vi "Top-Level.vi"() -> ()   [LabVIEW 2011]
uses:
  <vilib>/Platform/TimedLoop/XDataNode/timing_clust.ctl
  <vilib>/Platform/TimedLoop/XDataNode/nitl_modes.ctl
  <vilib>/Platform/TimedLoop/XDataNode/wakeup.ctl
  <vilib>/rvi/eio/common/nirviEmuTemplateMethod_errors.vi
  <vilib>/eio/EIONode/EIONode.xnode
  <vilib>/Platform/TimedLoop/XDataNode/XDataNode.xnode
  <vilib>/Platform/TimedLoop/XDataNode/XDNodeRunTimeDep.lvlib
panel:
  in  "manual steering":bool
  out "Velocity counts":u32
  out "Write error?":bool
  out "Read Error?":bool
  out "CS?":bool
  out "Indicator D":u32 format="%08x"
  out "Indicator C":u32 format="%08x"
  out "Indicator B":u32 format="%08x"
  out "Indicator A":u32 format="%08x"
  out "AI3":u32 format="%08x"
  out "AI2":u32 format="%08x"
  out "AI1":u32 format="%08x"
  out "AI0":u32 format="%08x"
  in  "Enable AI15":bool
  out "AI15":u16 format="%04d"
  in  "Enable AI14":bool
  out "AI14":u16 format="%04d"
  in  "Enable AI13":bool
  out "AI13":u16 format="%04d"
  in  "Enable AI12":bool
  out "AI12":u16 format="%04d"
  in  "Enable AI11":bool
  out "AI11":u16 format="%04d"
  in  "Enable AI10":bool
  out "AI10":u16 format="%04d"
  in  "Enable AI9":bool
  out "AI9":u16 format="%04d"
  in  "Enable AI8":bool
  out "AI8":u16 format="%04d"
  in  "Enable AI7":bool
  out "AI7":u16 format="%04d"
  in  "Enable AI6":bool
  out "AI6":u16 format="%04d"
  in  "Enable AI5":bool
  out "AI5":u16 format="%04d"
  in  "Enable AI4":bool
  out "AI4":u16 format="%04d"
  in  "Enable AI3":bool
  out "AI3":u16 format="%04d"
  in  "Enable AI2":bool
  out "AI2":u16 format="%04d"
  in  "Enable AI1":bool=TRUE
  out "AI1":u16 format="%04d"
  in  "Enable AI0":bool=TRUE
  out "AI0":u16 format="%04d"
  in  "ADC Run":bool=TRUE
  out "ADC Channel List":u16 format="%016b"
  in  "ADC Reset":bool
  out "Steering ON 1e-7s":u32
  out "Go Duty":u8
  out "Go Frequency":u16
  out "microblaze\\xps_gpio_0_GPIO_IO_O_pin 2":i32
  in  "manual throttle":bool
  out "Brake":bool
  out "Reverse":bool
  out "Enable":bool
  in  "uBlaze Reset":bool
  out "PWM0 period (cycles)":u32=400000
  out "PWM0 duty (cycles)":u32=80000
  in  "Clock Frequency (Hz)":u32=40000000
  out "PWM1 period(cycles)":u32=400000
  out "PWM1 duty (cycles)":u32=80000
  in  "PWM0 frequency (Hz)":u16
  in  "PWM0 duty (100*%)":u16
  in  "PWM1 frequency (Hz)":u16
  in  "PWM1 duty (100*%)":u16
  out "Steering period (cycles)":u32=400000
  out "Steering duty (cycles)":u32=80000
  out "GO period (cycles)":u32=400000
  out "GO duty (cycles)":u32=80000
  in  "Steering frequency (Hz)":u16=50
  in  "Steering ON 1e-7s":u32=8
  in  "GO frequency (Hz)":u16=1000
  in  "GO duty (100*%)":u16
  # "uBlaze Front Panel"
  # "ADC"
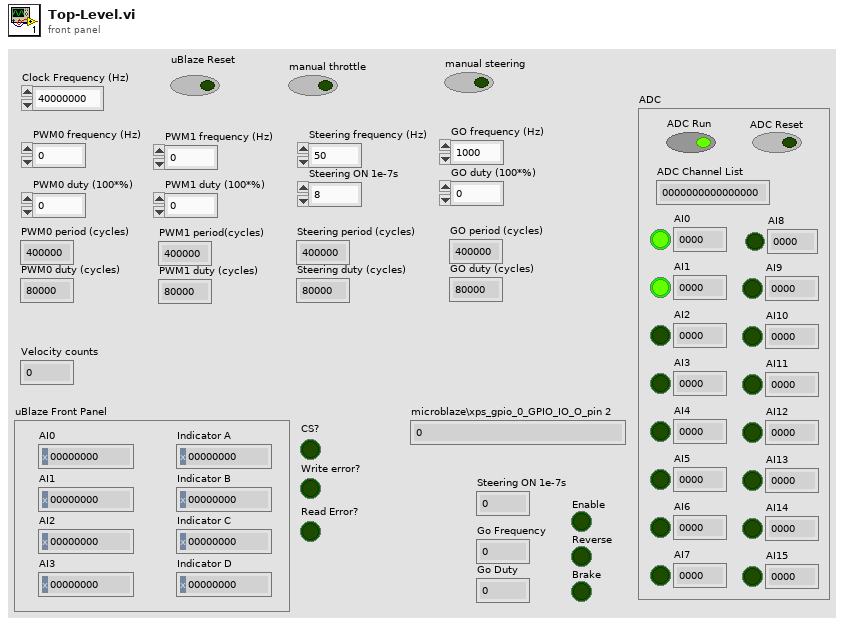
[diagram p1: front panel]
types:
  T1 = typedef "XDNodeRunTimeDep.lvlib/timing_clust.ctl" = cluster{"Expected End [f-1]":u64, "Actual End [f-1]":u64, "Finished Late? [f-1]":bool, "Expected End [i-1]":u64, "Actual End [i-1]":u64, "Finished Late? [i-1]":bool, "Expected Start [i]":u64, "Actual Start [i]":u64, "Expected Start [f]":u64, "Actual Start [f]":u64, "Source Name":string, "Structure Name":string, "Period":i64, "Deadline":i64, "Offset":i64, "Start":i64, "Priority":i32, "Timeout":i32, "Mode":T2, "Wakeup Reason":T3, "Error":errorcluster, "Source Type":string, "Secondary Source Type":string, "Global End Time":u64, "Global Start Time":u64, "Frame Duration":u64, "Iteration Duration":u64, "Assigned CPU":i32, "I/O Scan Engine Mode":u32}
  T2 = typedef "XDNodeRunTimeDep.lvlib/nitl_modes.ctl" = enum32{"No Change", "Process missed periods, maintain original phase", "Discard missed periods, maintain original phase", "Process missed periods, ignore original phase", "Discard missed periods, ignore original phase"}
  T3 = typedef "XDNodeRunTimeDep.lvlib/wakeup.ctl" = enum32{"Normal", "Aborted", "Asynchronous wakeup", "Timing source error", "Timed loop error", "Timeout"}
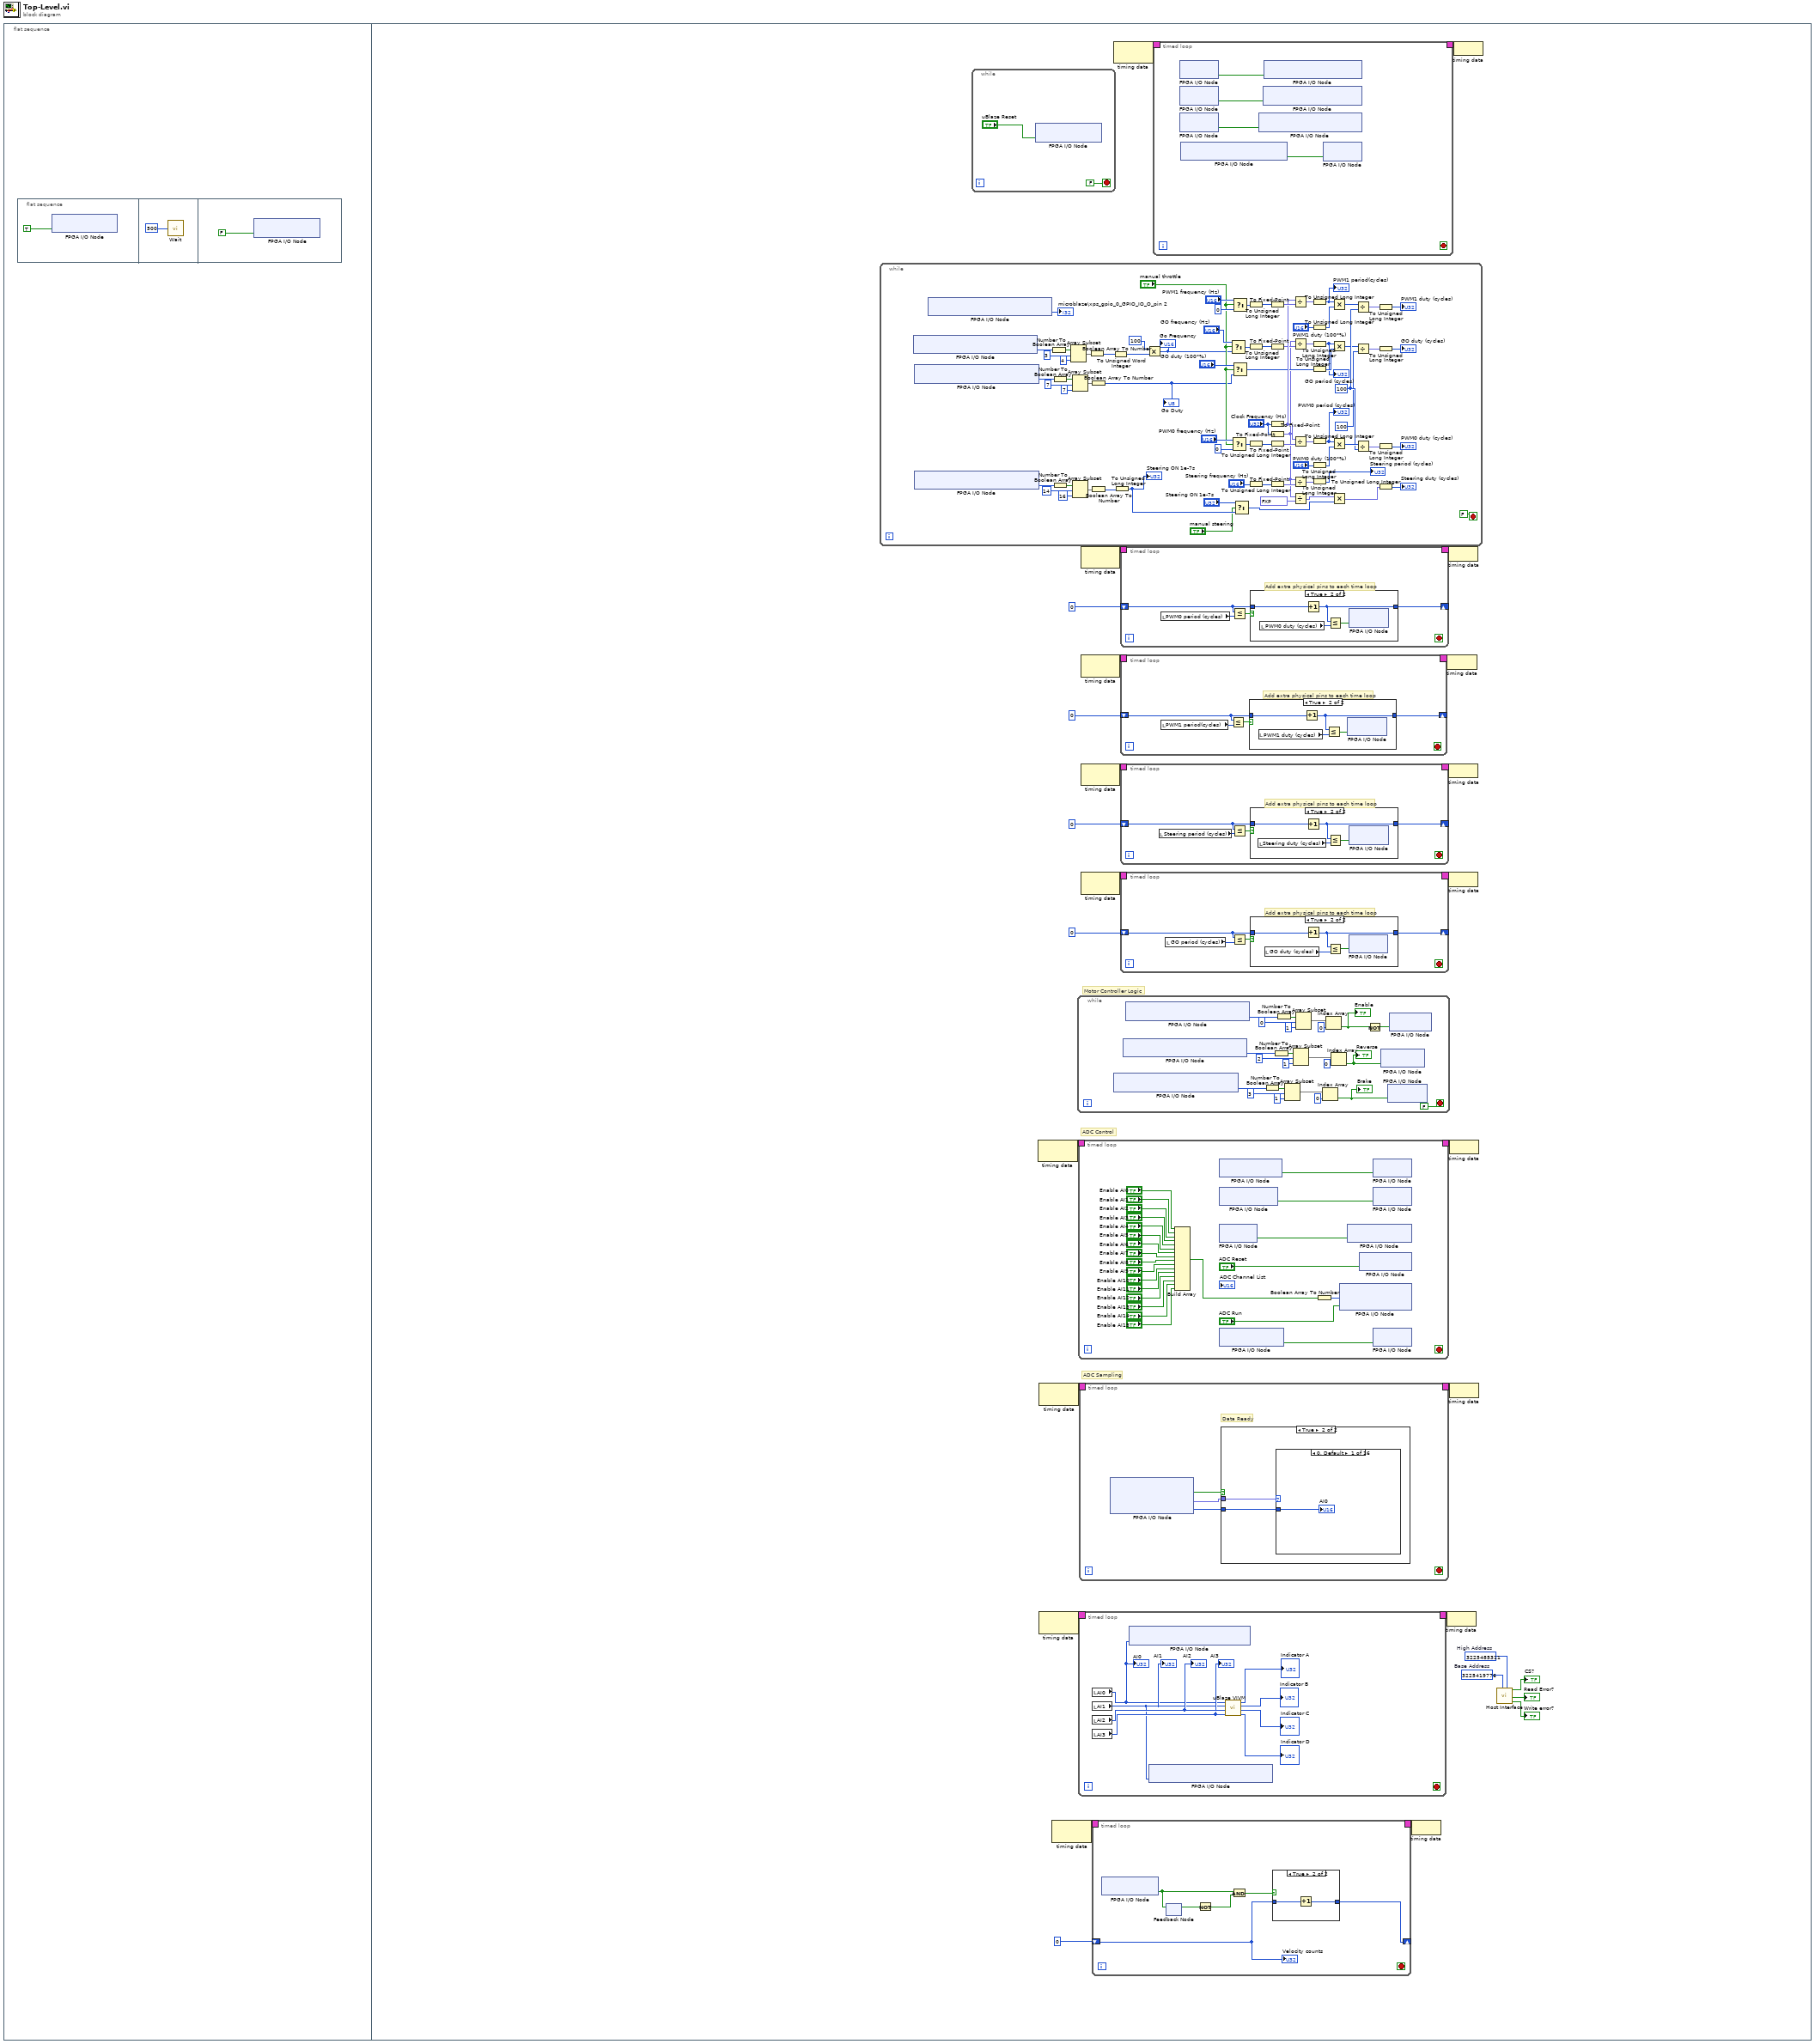
[diagram p0: block diagram]
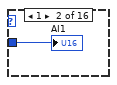
[diagram p4: hidden frame]
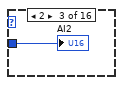
[diagram p5: hidden frame]
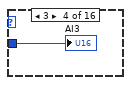
[diagram p6: hidden frame]
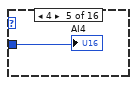
[diagram p7: hidden frame]
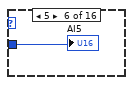
[diagram p8: hidden frame]
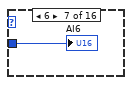
[diagram p9: hidden frame]
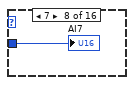
[diagram p10: hidden frame]
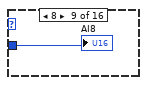
[diagram p11: hidden frame]
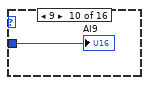
[diagram p12: hidden frame]
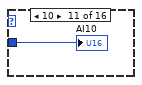
[diagram p13: hidden frame]
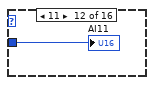
[diagram p14: hidden frame]
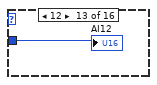
[diagram p15: hidden frame]
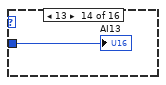
[diagram p16: hidden frame]
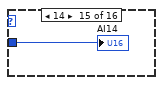
[diagram p17: hidden frame]
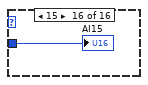
[diagram p18: hidden frame]
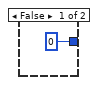
[diagram p19: hidden frame]
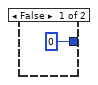
[diagram p20: hidden frame]
diagram:
  n1 = flat-sequence {
    frame #0 {
      n2 = flat-sequence {
        frame #0 {
          n3 = xnode "FPGA I/O Node"("microblaze\\reset"=TRUE ("Component-Level IP\\fpga_0_rst_1_sys_rst_pin")) -> ()  [unwired: 1 in, 1 out]
        }
        frame #1 {
          n4 = call "Wait"("Count(mSec)"=u32 500) -> ()  [unwired: 1 out]
        }
        frame #2 {
          n5 = xnode "FPGA I/O Node"("microblaze\\reset"=FALSE ("Component-Level IP\\fpga_0_rst_1_sys_rst_pin")) -> ()  [unwired: 1 in, 1 out]
        }
      }
    }
    frame #1 {
      w12 = u32 3225485311  # High Address
      w13 = u32 3225419776  # Base Address
      # "ADC Sampling"
      # "ADC Control"
      # "Motor Controller Logic"
      n6 = while {
        stop <- FALSE stop-if-true
        w191 = u32 100 ("y")
        n7 = xnode "FPGA I/O Node"() -> ("microblaze\\xps_gpio_0_GPIO_IO_O_pin"=w156:i32)  [unwired: 1 in, 1 out]
        n8 = xnode "FPGA I/O Node"() -> ("microblaze\\xps_gpio_0_GPIO_IO_O_pin"=w150:i32)  [unwired: 1 in, 1 out]
        n9 = xnode "FPGA I/O Node"() -> ("microblaze\\xps_gpio_0_GPIO_IO_O_pin"=w151:i32)  [unwired: 1 in, 1 out]
        n10 = xnode "FPGA I/O Node"() -> ("microblaze\\xps_gpio_0_GPIO_IO_O_pin"=→"microblaze\\xps_gpio_0_GPIO_IO_O_pin 2":i32)  [unwired: 1 in, 1 out]
        n11 = Number To Boolean Array(number=w156) -> (Boolean array=w160:bool[])
        n12 = Number To Boolean Array(number=w150) -> (Boolean array=w146:bool[])
        n13 = Number To Boolean Array(number=w151) -> (Boolean array=w155:bool[])
        n14 = Array Subset(array=w160, index=3, length=4) -> (w159:bool[])
        n15 = Array Subset(array=w146, index=7, length=7) -> (w147:bool[])
        n16 = Array Subset(array=w155, index=14, length=16) -> (w154:bool[])
        n17 = Boolean Array To Number(Boolean array=w159) -> (number=w143:u8)
        n18 = Boolean Array To Number(Boolean array=w147) -> (number=w145:u8)
        "Go Duty" <- w145
        n19 = Boolean Array To Number(Boolean array=w154) -> (number=w135:u16)
        n20 = To Unsigned Word Integer(number=w143) -> (unsigned 16bit integer=w142:u16)
        n21 = To Unsigned Long Integer(number=w135) -> (unsigned 32bit integer=w134:u32)
        "Steering ON 1e-7s" <- w134
        n22 = Multiply(x=u16 100, y=w142) -> (x*y=w162:u16)
        "Go Frequency" <- w162
        n23 = Select(t="GO frequency (Hz)", s="manual throttle", f=w162) -> (s? t:f=w174:u16)
        n24 = Select(t="PWM0 frequency (Hz)", s="manual throttle", f=u16 0) -> (s? t:f=w172:u16)
        n25 = Select(t="GO duty (100*%)", s="manual throttle", f=w145) -> (s? t:f=w170:u16)
        n26 = Select(t="PWM1 frequency (Hz)", s="manual throttle", f=u16 0) -> (s? t:f=w176:u16)
        n27 = Select(t="Steering ON 1e-7s", s="manual steering", f=w134) -> (s? t:f=w137:u32)
        n28 = To Unsigned Long Integer(number=w176) -> (unsigned 32bit integer=w199:u32)
        n29 = To Unsigned Long Integer(number=w174) -> (unsigned 32bit integer=w184:u32)
        n30 = To Unsigned Long Integer(number=w172) -> (unsigned 32bit integer=w203:u32)
        n31 = To Unsigned Long Integer(number="Steering frequency (Hz)") -> (unsigned 32bit integer=w186:u32)
        n32 = To Fixed-Point(number=w199) -> (fixed-point=w198:fxp<+,32,32>)  [unwired: 1 out]
        n33 = To Fixed-Point(number=w184) -> (fixed-point=w183:fxp<+,32,32>)  [unwired: 1 out]
        n34 = To Fixed-Point(number="Clock Frequency (Hz)") -> (fixed-point=w192:fxp<+,32,32>)  [unwired: 1 out]
        n35 = To Fixed-Point(number="Clock Frequency (Hz)") -> (fixed-point=w141:fxp<+,32,32>)  [unwired: 1 out]
        n36 = To Fixed-Point(number=w203) -> (fixed-point=w204:fxp<+,32,32>)  [unwired: 1 out]
        n37 = To Fixed-Point(number=w186) -> (fixed-point=w187:fxp<+,32,32>)  [unwired: 1 out]
        n38 = Divide(x=w192, y=w198) -> (x/y=w193:fxp<+,32,33>)
        n39 = Divide(x=w141, y=w183) -> (x/y=w178:fxp<+,32,33>)
        n40 = Divide(x=w192, y=w204) -> (x/y=w209:fxp<+,32,33>)
        n41 = Divide(x=w141, y=w187) -> (x/y=w189:fxp<+,32,33>)
        n42 = Divide(x=w141, y=fxp<+,32,32> 10000000.0) -> (x/y=w138:fxp<+,64,32>)
        n43 = To Unsigned Long Integer(number=w193) -> (unsigned 32bit integer=w194:u32)
        "PWM1 period(cycles)" <- w194
        n44 = To Unsigned Long Integer(number="PWM1 duty (100*%)") -> (unsigned 32bit integer=w200:u32)
        n45 = To Unsigned Long Integer(number=w178) -> (unsigned 32bit integer=w179:u32)
        "GO period (cycles)" <- w179
        n46 = To Unsigned Long Integer(number=w170) -> (unsigned 32bit integer=w185:u32)
        n47 = To Unsigned Long Integer(number=w209) -> (unsigned 32bit integer=w208:u32)
        "PWM0 period (cycles)" <- w208
        n48 = To Unsigned Long Integer(number="PWM0 duty (100*%)") -> (unsigned 32bit integer=w201:u32)
        n49 = To Unsigned Long Integer(number=w189) -> (unsigned 32bit integer=→"Steering period (cycles)":u32)
        n50 = Multiply(x=w194, y=w200) -> (x*y=w195:u32)
        n51 = Multiply(x=w179, y=w185) -> (x*y=w180:u32)
        n52 = Multiply(x=w208, y=w201) -> (x*y=w207:u32)
        n53 = Multiply(x=w138, y=w137) -> (x*y=w136:fxp<+,64,64>)
        n54 = Divide(x=w195, y=w191) -> (x/y=w196:fxp<+,32,33>)
        n55 = Divide(x=w180, y=u32 100) -> (x/y=w181:fxp<+,32,33>)
        n56 = Divide(x=w207, y=w191) -> (x/y=w206:fxp<+,32,33>)
        n57 = To Unsigned Long Integer(number=w196) -> (unsigned 32bit integer=→"PWM1 duty (cycles)":u32)
        n58 = To Unsigned Long Integer(number=w181) -> (unsigned 32bit integer=→"GO duty (cycles)":u32)
        n59 = To Unsigned Long Integer(number=w206) -> (unsigned 32bit integer=→"PWM0 duty (cycles)":u32)
        n60 = To Unsigned Long Integer(number=w136) -> (unsigned 32bit integer=→"Steering duty (cycles)":u32)
      }
      n61 = while {
        stop <- FALSE stop-if-true
        n62 = xnode "FPGA I/O Node"("microblaze\\reset"="uBlaze Reset") -> ()  [unwired: 1 in, 1 out]
      }
      n63 = node-c288() -> (w17:T1)  [unwired: 1 in]
      n64 = node-c288() -> (w8:T1)  [unwired: 1 in]
      n65 = node-c288() -> (w15:T1)  [unwired: 1 in]
      n66 = node-c288() -> (w6:T1)  [unwired: 1 in]
      n67 = while {
        stop <- FALSE stop-if-true
        n68 = xnode "FPGA I/O Node"() -> ("microblaze\\xps_gpio_0_GPIO_IO_O_pin"=w119:i32)  [unwired: 1 in, 1 out]
        n69 = xnode "FPGA I/O Node"() -> ("microblaze\\xps_gpio_0_GPIO_IO_O_pin"=w126:i32)  [unwired: 1 in, 1 out]
        n70 = xnode "FPGA I/O Node"() -> ("microblaze\\xps_gpio_0_GPIO_IO_O_pin"=w129:i32)  [unwired: 1 in, 1 out]
        n71 = Number To Boolean Array(number=w119) -> (Boolean array=w122:bool[])
        n72 = Number To Boolean Array(number=w126) -> (Boolean array=w123:bool[])
        n73 = Number To Boolean Array(number=w129) -> (Boolean array=w132:bool[])
        n74 = Array Subset(array=w122, index=3, length=1) -> (w116:bool[])
        n75 = Array Subset(array=w123, index=2, length=1) -> (w117:bool[])
        n76 = Array Subset(array=w132, index=0, length=1) -> (w113:bool[])
        n77 = Index Array(array=w116, index=0) -> (element=w114:bool)
        "Brake" <- w114
        n78 = Index Array(array=w113, index=0) -> (element=w111:bool)
        "Enable" <- w111
        n79 = Index Array(array=w117, index=0) -> (element=w115:bool)
        "Reverse" <- w115
        n80 = Not(x=w111) -> (.not. x?=w112:bool)
        n81 = xnode "FPGA I/O Node"("REVERSE"=w115) -> ()  [unwired: 1 in, 1 out]
        n82 = xnode "FPGA I/O Node"("BRAKE"=w114) -> ()  [unwired: 1 in, 1 out]
        n83 = xnode "FPGA I/O Node"("ENABLE"=w112) -> ()  [unwired: 1 in, 1 out]
      }
      n84 = timed-loop {
        timing: w17 -> [_]
        timing-out: [_] -> w16
        stop <- _ stop-if-true
        n85 = Build Array("Enable AI0", "Enable AI1", "Enable AI2", "Enable AI3", "Enable AI4", "Enable AI5", "Enable AI6", "Enable AI7", "Enable AI8", "Enable AI9", "Enable AI10", "Enable AI11", "Enable AI12", "Enable AI13", "Enable AI14", "Enable AI15") -> (w98:bool[])
        n86 = xnode "FPGA I/O Node"() -> ("ADC\\aaispics_n"=w100:bool)  [unwired: 1 in, 1 out]
        n87 = xnode "FPGA I/O Node"() -> ("ADC\\aaispiclk"=w101:bool)  [unwired: 1 in, 1 out]
        n88 = xnode "FPGA I/O Node"() -> ("SDO"=w102:bool)  [unwired: 1 in, 1 out]
        n89 = xnode "FPGA I/O Node"() -> ("ADC\\aaispimosi"=w103:bool)  [unwired: 1 in, 1 out]
        n90 = Boolean Array To Number(Boolean array=w98) -> (number=w99:u16)
        n91 = xnode "FPGA I/O Node"("ADC\\caichannellist"=w99, "ADC\\cairun"="ADC Run") -> ()  [unwired: 2 in, 2 out]
        n92 = xnode "FPGA I/O Node"("ADC\\aaispimiso"=w102) -> ()  [unwired: 1 in, 1 out]
        n93 = xnode "FPGA I/O Node"("ADC\\areset"="ADC Reset") -> ()  [unwired: 1 in, 1 out]
        n94 = xnode "FPGA I/O Node"("CS"=w100) -> ()  [unwired: 1 in, 1 out]
        n95 = xnode "FPGA I/O Node"("SCLK"=w101) -> ()  [unwired: 1 in, 1 out]
        n96 = xnode "FPGA I/O Node"("SDI"=w103) -> ()  [unwired: 1 in, 1 out]
      }
      n97 = timed-loop {
        timing: w8 -> [_]
        timing-out: [_] -> w7
        stop <- _ stop-if-true
        n98 = local read "AI0"() -> (w45:u16)
        "AI0" <- w45
        n99 = local read "AI1"() -> (w46:u16)
        "AI1" <- w46
        n100 = local read "AI2"() -> (w48:u16)
        "AI2" <- w48
        n101 = local read "AI3"() -> (w47:u16)
        "AI3" <- w47
        n102 = xnode "FPGA I/O Node"("microblaze\\xps_gpio_1_GPIO_IO_I_pin"=w45) -> ()  [unwired: 1 in, 1 out]
        n103 = xnode "FPGA I/O Node"("microblaze\\xps_gpio_1_GPIO2_IO_I_pin"=w46) -> ()  [unwired: 1 in, 1 out]
        n104 = call "uBlaze VIVM.vi"("Control D (+0x000C)"=w47, "Control C (+0x0008)"=w48, "Control B (+0x0004)"=w46, "Control A (+0x0000)"=w45) -> ("Indicator D (+0x001C)"=→"Indicator D":u32, "Indicator C (+0x0018)"=→"Indicator C":u32, "Indicator B (+0x0014)"=→"Indicator B":u32, "Indicator A (+0x0010)"=→"Indicator A":u32)  [unwired: 4 in]
      }
      n105 = timed-loop {
        timing: w15 -> [_]
        timing-out: [_] -> w14
        stop <- _ stop-if-true
        # "Data Ready"
        n106 = xnode "FPGA I/O Node"() -> ("ADC\\caidataready"=w59:bool, "ADC\\caicurrentchannel"=w57:fxp<+,4,4>, "ADC\\caidataout"=w58:u16)  [unwired: 3 in, 3 out]
        n107 = case shown="True" w59 {
          tunnel: w57 -> [_ w61]
          tunnel: w58 -> [_ w60]
          frame False {
          }
          frame True {
            n108 = case shown="0, Default" w61 {
              tunnel: w60 -> [w62 w63 w64 w65 w66 w67 w68 w69 w70 w71 w72 w73 w74 w75 w76 w77]
              frame 0, Default {
                "AI0" <- w62
              }
              frame 1 {
                "AI1" <- w63
              }
              frame 2 {
                "AI2" <- w64
              }
              frame 3 {
                "AI3" <- w65
              }
              frame 4 {
                "AI4" <- w66
              }
              frame 5 {
                "AI5" <- w67
              }
              frame 6 {
                "AI6" <- w68
              }
              frame 7 {
                "AI7" <- w69
              }
              frame 8 {
                "AI8" <- w70
              }
              frame 9 {
                "AI9" <- w71
              }
              frame 10 {
                "AI10" <- w72
              }
              frame 11 {
                "AI11" <- w73
              }
              frame 12 {
                "AI12" <- w74
              }
              frame 13 {
                "AI13" <- w75
              }
              frame 14 {
                "AI14" <- w76
              }
              frame 15 {
                "AI15" <- w77
              }
            }
          }
        }
      }
      n109 = node-c288() -> (w29:T1)  [unwired: 1 out]
      n110 = node-c288() -> (w27:T1)  [unwired: 1 out]
      n111 = node-c288() -> (w25:T1)  [unwired: 1 out]
      n112 = node-c288() -> (w23:T1)  [unwired: 1 out]
      n113 = timed-loop {
        timing: w6 -> [_]
        timing-out: [_] -> w5
        shift-right: [w33] -> _
        shift-left: u32 0 -> [w32]
        stop <- _ stop-if-true
        n114 = xnode "FPGA I/O Node"() -> ("ENCODER_IN"=w35:bool)  [unwired: 1 in, 1 out]
        n115 = feedback-in #1(w35) -> ()
        n116 = feedback #1() -> (w36:bool)  [unwired: 1 in]
        n117 = Not(x=w36) -> (.not. x?=w37:bool)
        n118 = And(x=w35, y=w37) -> (x .and. y?=w34:bool)
        n119 = case shown="True" w34 {
          tunnel: w32 -> [w38 w40]
          tunnel: [w38 w39] -> w33
          frame False {
          }
          frame True {
            n120 = Increment(x=w40) -> (x+1=w39:u32)
          }
        }
        "Velocity counts" <- w32
      }
      n121 = node-c288() -> (w31:T1)  [unwired: 1 in]
      n122 = timed-loop {
        timing: w29 -> [_]
        timing-out: [_] -> w28
        shift-right: [w253] -> _
        shift-left: u32 0 -> [w254]
        stop <- _ stop-if-true
        # "Add extra physical pins to each time loop"
        n123 = local read "PWM0 period (cycles)"() -> (w252:u32)
        n124 = Less Or Equal?(x=w254, y=w252) -> (x <= y?=w255:bool)
        n125 = case shown="True" w255 {
          tunnel: w254 -> [_ w260]
          tunnel: [i16 0 w259] -> w253
          frame False {
          }
          frame True {
            n126 = local read "PWM0 duty (cycles)"() -> (w258:u32)
            n127 = Increment(x=w260) -> (x+1=w259:u32)
            n128 = Less Or Equal?(x=w259, y=w258) -> (x <= y?=w257:bool)
            n129 = xnode "FPGA I/O Node"("PWM0"=w257) -> ()  [unwired: 1 in, 1 out]
          }
        }
      }
      n130 = timed-loop {
        timing: w27 -> [_]
        timing-out: [_] -> w26
        shift-right: [w240] -> _
        shift-left: u32 0 -> [w241]
        stop <- _ stop-if-true
        # "Add extra physical pins to each time loop"
        n131 = local read "PWM1 period(cycles)"() -> (w239:u32)
        n132 = Less Or Equal?(x=w241, y=w239) -> (x <= y?=w242:bool)
        n133 = case shown="True" w242 {
          tunnel: w241 -> [_ w247]
          tunnel: [i16 0 w246] -> w240
          frame False {
          }
          frame True {
            n134 = local read "PWM1 duty (cycles)"() -> (w245:u32)
            n135 = Increment(x=w247) -> (x+1=w246:u32)
            n136 = Less Or Equal?(x=w246, y=w245) -> (x <= y?=w244:bool)
            n137 = xnode "FPGA I/O Node"("PWM1"=w244) -> ()  [unwired: 1 in, 1 out]
          }
        }
      }
      n138 = timed-loop {
        timing: w25 -> [_]
        timing-out: [_] -> w24
        shift-right: [w227] -> _
        shift-left: u32 0 -> [w228]
        stop <- _ stop-if-true
        # "Add extra physical pins to each time loop"
        n139 = local read "Steering period (cycles)"() -> (w226:u32)
        n140 = Less Or Equal?(x=w228, y=w226) -> (x <= y?=w229:bool)
        n141 = case shown="True" w229 {
          tunnel: w228 -> [_ w234]
          tunnel: [i16 0 w233] -> w227
          frame False {
          }
          frame True {
            n142 = local read "Steering duty (cycles)"() -> (w232:u32)
            n143 = Increment(x=w234) -> (x+1=w233:u32)
            n144 = Less Or Equal?(x=w233, y=w232) -> (x <= y?=w231:bool)
            n145 = xnode "FPGA I/O Node"("PWM2"=w231) -> ()  [unwired: 1 in, 1 out]
          }
        }
      }
      n146 = timed-loop {
        timing: w23 -> [_]
        timing-out: [_] -> w22
        shift-right: [w214] -> _
        shift-left: u32 0 -> [w215]
        stop <- _ stop-if-true
        # "Add extra physical pins to each time loop"
        n147 = local read "GO period (cycles)"() -> (w213:u32)
        n148 = Less Or Equal?(x=w215, y=w213) -> (x <= y?=w216:bool)
        n149 = case shown="True" w216 {
          tunnel: w215 -> [_ w221]
          tunnel: [i16 0 w220] -> w214
          frame False {
          }
          frame True {
            n150 = local read "GO duty (cycles)"() -> (w219:u32)
            n151 = Increment(x=w221) -> (x+1=w220:u32)
            n152 = Less Or Equal?(x=w220, y=w219) -> (x <= y?=w218:bool)
            n153 = xnode "FPGA I/O Node"("GO"=w218) -> ()  [unwired: 1 in, 1 out]
          }
        }
      }
      n154 = timed-loop {
        timing: w31 -> [_]
        timing-out: [_] -> w30
        stop <- _ stop-if-true
        n155 = xnode "FPGA I/O Node"() -> ("TCK"=w268:bool)  [unwired: 1 in, 1 out]
        n156 = xnode "FPGA I/O Node"() -> ("TMS"=w267:bool)  [unwired: 1 in, 1 out]
        n157 = xnode "FPGA I/O Node"() -> ("TDI"=w266:bool)  [unwired: 1 in, 1 out]
        n158 = xnode "FPGA I/O Node"() -> ("microblaze\\mdm_0_extTDO_pin"=w265:bool)  [unwired: 1 in, 1 out]
        n159 = xnode "FPGA I/O Node"("microblaze\\mdm_0_extTDI_pin"=w266) -> ()  [unwired: 1 in, 1 out]
        n160 = xnode "FPGA I/O Node"("microblaze\\mdm_0_TMS_pin"=w267) -> ()  [unwired: 1 in, 1 out]
        n161 = xnode "FPGA I/O Node"("microblaze\\mdm_0_TCK_pin"=w268) -> ()  [unwired: 1 in, 1 out]
        n162 = xnode "FPGA I/O Node"("TDO"=w265) -> ()  [unwired: 1 in, 1 out]
      }
      n163 = node-c288(w5) -> ()
      n164 = node-c288(w7) -> ()
      n165 = node-c288(w26) -> ()
      n166 = node-c288(w28) -> ()
      n167 = node-c288(w24) -> ()
      n168 = node-c288(w22) -> ()
      n169 = node-c288(w16) -> ()
      n170 = node-c288(w14) -> ()
      n171 = node-c288(w30) -> ()
      n172 = call "Host Interface.vi"("High Address"=w12, "Base Address"=w13) -> ("Write error?"=→"Write error?":bool, "Read Error?"=→"Read Error?":bool, "CS?"=→"CS?":bool)  [unwired: 7 in]
    }
  }
